vi "Setup transport options.vi"(8 "error in (no error)":errorcluster, 11 "WAMP Client in":refnum<class "WAMP Client.lvclass">) -> (0 "error out":errorcluster, 3 "WAMP Client out":refnum<class "WAMP Client.lvclass">)   [LabVIEW 2020, in "wamplv.lvlib" / "WAMP Client.lvclass"]
uses:
  WAMP Client.lvclass
  WAMP Client.lvclass/WAMP Client.ctl
  Private/Comm Handlers/Websocket Handler/Websocket Handler.lvclass
  C:/local/wamplv/Private/Comm Handlers/ICommHandler/ICommHandler.lvclass
  C:/local/wamplv/Private/Comm Handlers/CommHandlerBase/CommHandlerBase.lvclass
  C:/local/wamplv/Private/Comm Handlers/Websocket Handler/Websocket Handler.lvclass
  Private/Comm Handlers/ICommHandler/ICommHandler.lvclass
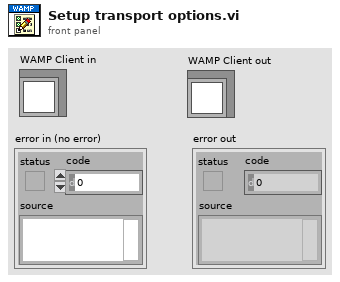
[diagram p1: front panel]
types:
  T1 = typedef "wamplv.lvlib/WAMP Client.lvclass/Transport Type.ctl" = enum16{"WebSocket", "RawSocket TCP"}
  T2 = typedef "wamplv.lvlib/Websocket Handler.lvclass/Options.ctl" = cluster{"Send Headers":T3[]}
  T3 = typedef "wamplv.lvlib/Websocket Handler.lvclass/Headers.ctl" = cluster{"Name":string, "Value":string}
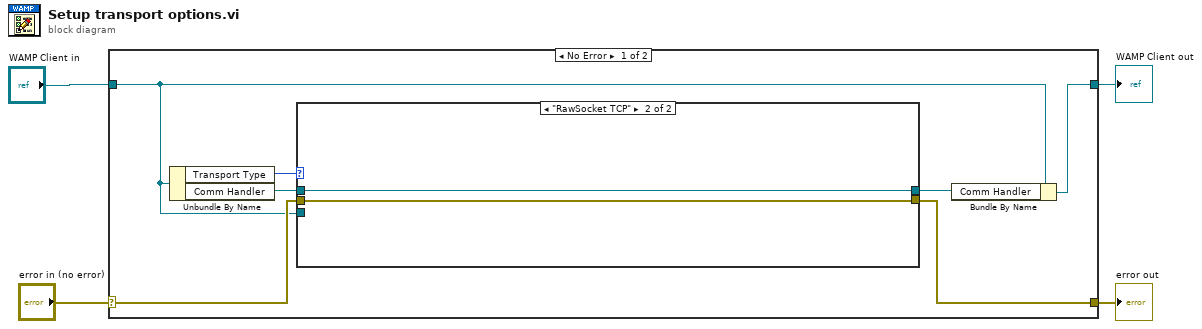
[diagram p0: block diagram]
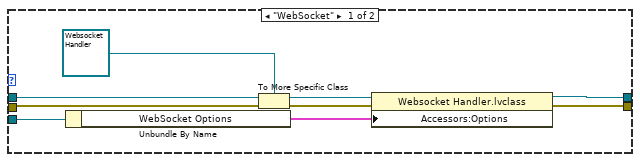
[diagram p2: hidden frame]
diagram:
  n1 = case shown="No Error" "error in (no error)" {
    selector: "error in (no error)" -> [w11 w23]
    tunnel: [w10 w23] -> w3
    tunnel: [w6 w24] -> w1
    tunnel: "WAMP Client in" -> [w8 w24]
    frame No Error {
      n2 = Unbundle By Name(w8) -> ("Transport Type"=w9:T1, "Comm Handler"=w5:refnum<class "ICommHandler.lvclass">)
      n3 = case shown="\"RawSocket TCP\"" w9 {
        tunnel: w11 -> [w19 w22]
        tunnel: [w15 w22] -> w10
        tunnel: w8 -> [w14 _]
        tunnel: [w13 w21] -> w7
        tunnel: w5 -> [w12 w21]
        frame "WebSocket" {
          n4 = Unbundle By Name(w14) -> ("WebSocket Options"=w16:T2)
          n5 = To More Specific Class(target class=refnum<class "Websocket Handler.lvclass"> refnum ("wamplv.lvlib:Websocket Handler.lvclass"), reference=w12, error in=w19) -> (specific class reference=w18:refnum<class "Websocket Handler.lvclass">, error out=w17:errorcluster)
          n6 = property class="Websocket Handler.lvclass"(reference=w18, error in=w17, "Accessors:Options"=w16) -> (reference out=w13:refnum<class "Websocket Handler.lvclass">, error out=w15:errorcluster)
        }
        frame "RawSocket TCP" {
        }
      }
      n7 = Bundle By Name(cluster=w8, "Comm Handler"=w7) -> (w6:refnum<class "WAMP Client.lvclass">)
    }
    frame Error {
    }
  }
  "error out" <- w3
  "WAMP Client out" <- w1
